vi "get_libraryBlacklist.vi"(0 "Host_Reference":refnum<class "HGF_Reference.lvclass">, 2 "timeout in ms (-1)":i32=-1, 5 "error in (no error)":errorcluster) -> (14 "dup Host_Reference":refnum<class "HGF_Reference.lvclass">, 16 "Library Blacklist":string[](array[string]), 19 "error out":errorcluster)   [LabVIEW 2009, in "MoAgSy.lvlib" / "MoAgSy_Host.lvclass"]
doc: "<B>public</B> VI returns referenced Hosts library blacklist.\nAgents that are mebers of blacklisted libraries will not be started at this host system.\n\nF.Berck@gsi.de\nGSI Darmstadt 2009"
uses:
  MoAgSy_Host.lvclass
  HGF_BaseClasses/HGF_Reference/HGF_Reference.lvclass
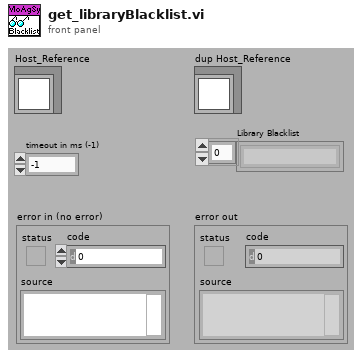
[diagram p1: front panel]
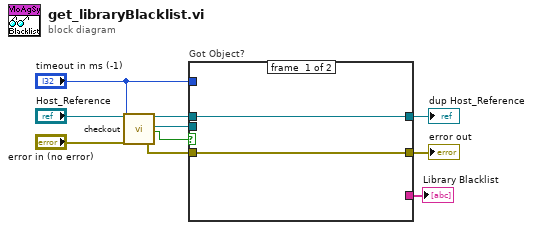
[diagram p0: block diagram]
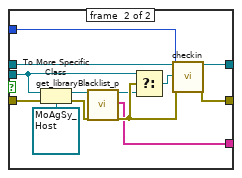
[diagram p2: hidden frame]
diagram:
  n1 = call "checkout.vi"("HGF_Reference"="Host_Reference", "timeout in ms (-1)"="timeout in ms (-1)", "error in (no error)"="error in (no error)") -> ("dup HGF_Reference"=w5:refnum<class "HGF_Reference.lvclass">, "Object"=w8:refnum<class>, "got object?"=w6:bool, "error out"=w9:errorcluster)  [unwired: 13 out]
  n2 = case "Got Object?" shown="True" w6 {
    tunnel: w9 -> [w11 w24]
    tunnel: w8 -> [_ w17]
    tunnel: w5 -> [w12 w22]
    tunnel: [w12 w21] -> w4
    tunnel: "timeout in ms (-1)" -> [_ w20]
    tunnel: [w11 w19] -> w2
    tunnel: [_ w13] -> w1
    frame #0 {
    }
    frame #1 {
      n3 = To More Specific Class(target class=refnum<class "MoAgSy_Host.lvclass"> refnum ("MoAgSy.lvlib:MoAgSy_Host.lvclass"), reference=w17, error in=w24) -> (specific class reference=w18:refnum<class "MoAgSy_Host.lvclass">, error out=w14:errorcluster)
      n4 = call "get_libraryBlacklist_p.vi"("MoAgSy_Host"=w18, "error in (no error)"=w14) -> ("dup MoAgSy_Host"=w15:refnum<class "MoAgSy_Host.lvclass">, "Library Blacklist"=w13:string[], "error out"=w25:errorcluster)  [unwired: 15 out]
      n5 = Select(t=w17, s=w25, f=w15) -> (s? t:f=w16:refnum<class>)
      n6 = call "checkin.vi"("HGF_Reference"=w22, "Object"=w16, "timeout /ms (-1)"=w20, "error in (no error)"=w25) -> ("dup HGF_Reference"=w21:refnum<class "HGF_Reference.lvclass">, "error out"=w19:errorcluster)  [unwired: 14 out]
    }
  }
  "dup Host_Reference" <- w4
  "error out" <- w2
  "Library Blacklist" <- w1
